vi "TRABAJO3.vi"() -> ()   [LabVIEW 2022 SP3]
panel:
  in  "Strings, Ciclos y Eventos":enum32{"EJERCICIO 1", "EJERCICIO 2"}(tab)
  out "SERIE FIBONACCI":string
  in  "LÍMITE SUPERIOR":dbl
  in  "?":bool
  out "ITERACIONES":dbl
  out "CONTADOR":dbl
  in  "?":bool
  in  "?":bool
  in  "?":bool
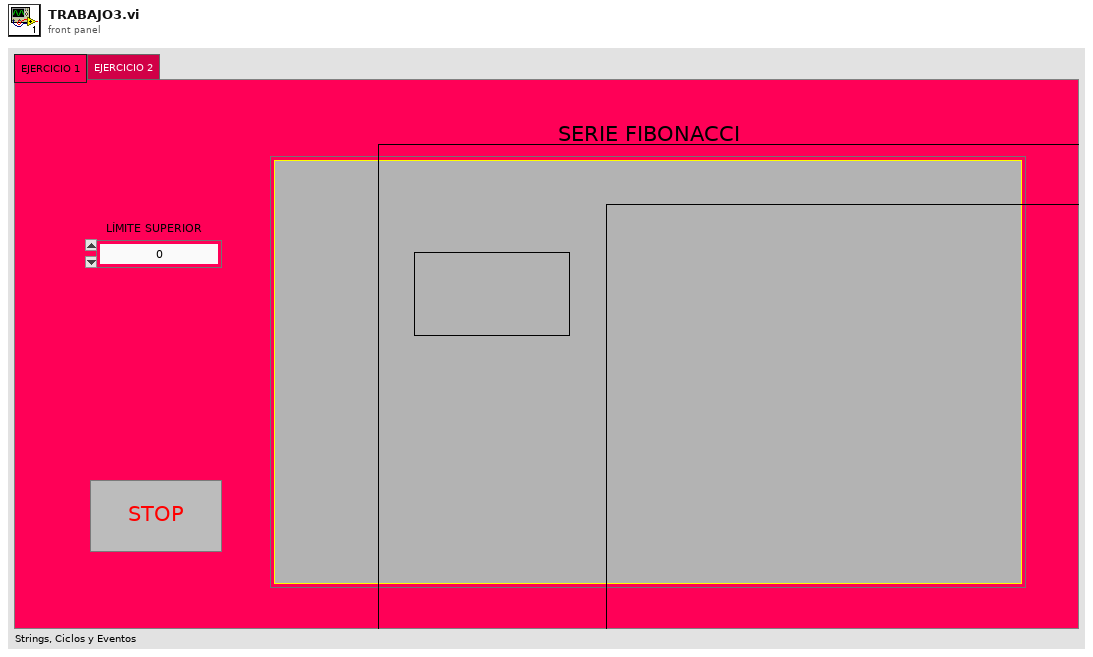
[diagram p1: front panel]
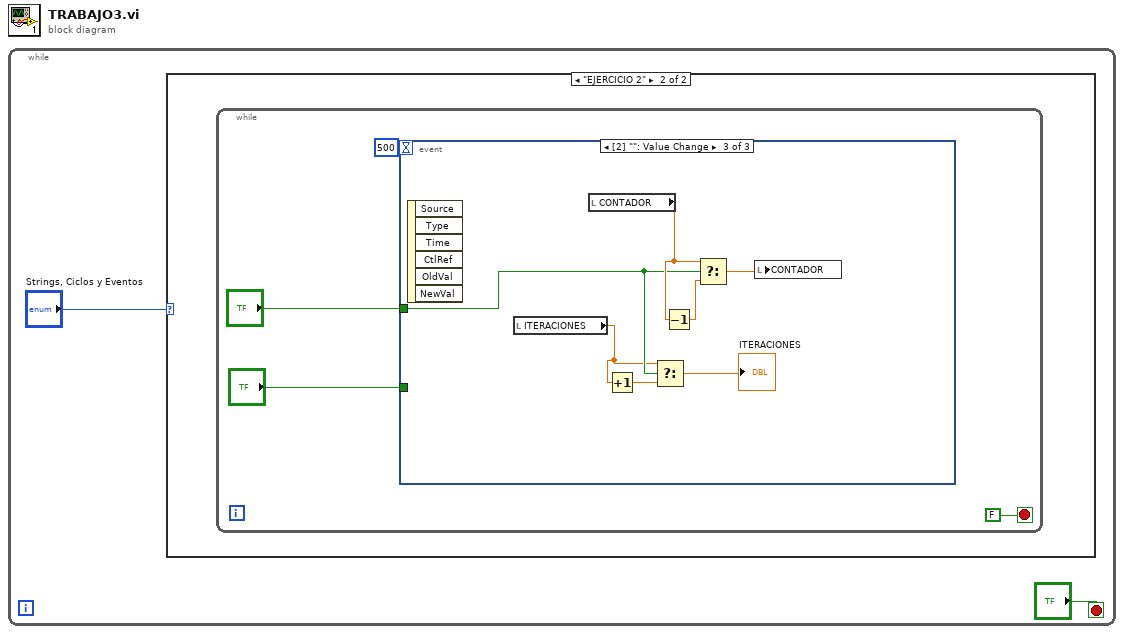
[diagram p0: block diagram]
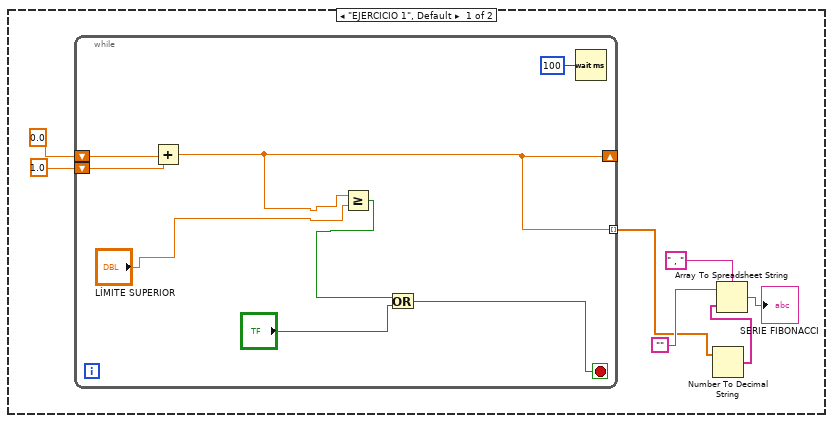
[diagram p2: hidden frame]
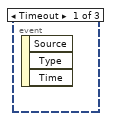
[diagram p3: hidden frame]
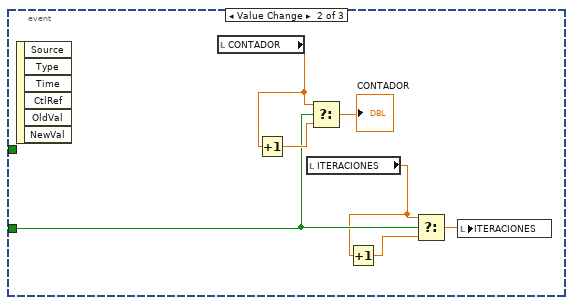
[diagram p4: hidden frame]
diagram:
  n1 = while {
    stop <- "?" stop-if-true
    n2 = case shown="\"EJERCICIO 2\"" "Strings, Ciclos y Eventos" {
      frame "EJERCICIO 1", Default {
        n3 = while {
          shift-right: [w12] -> _
          shift-left: 0.0 -> [w17]
          shift-left: 1.0 -> [w16]
          tunnel: [w12] -> w4 mode=indexing
          stop <- w14 stop-if-true
          n4 = Add(x=w17, y=w16) -> (x+y=w12:dbl)
          n5 = Greater Or Equal?(x=w12, y="LÍMITE SUPERIOR") -> (x >= y?=w10:bool)
          n6 = Or(x=w10, y="?") -> (x .or. y?=w14:bool)
          n7 = Wait (ms)(milliseconds to wait=u32 100) -> ()  [unwired: 1 out]
        }
        n8 = Number To Decimal String(number=w4) -> (decimal integer string=w3:string[])  [unwired: 1 in]
        n9 = Array To Spreadsheet String(delimiter (Tab)=" , ", array=w3, 3:"") -> (spreadsheet string=→"SERIE FIBONACCI":string)
      }
      frame "EJERCICIO 2" {
        n10 = while {
          stop <- FALSE stop-if-true
          n11 = event shown="[2] \"\": Value Change" {
            selector: _ -> [_ _ _]
            dyn-events: _ -> [_ _ _]
            timeout: 500 -> [_ _ _]
            tunnel: "?" -> [_ _ w31]
            tunnel: "?" -> [_ w24 _]
            event Timeout {
              n12 = event-data() -> ()  [unwired: 1 in, 3 out]
            }
            event Value Change {
              n13 = event-data() -> ()  [unwired: 1 in, 6 out]
              n14 = local read "CONTADOR"() -> (w26:dbl)
              n15 = Increment(x=w26) -> (x+1=w27:dbl)
              n16 = local read "ITERACIONES"() -> (w22:dbl)
              n17 = Select(t=w26, s=w24, f=w27) -> (s? t:f=→"CONTADOR":dbl)
              n18 = Increment(x=w22) -> (x+1=w23:dbl)
              n19 = Select(t=w22, s=w24, f=w23) -> (s? t:f=w25:dbl)
              n20 = local write "ITERACIONES"(w25) -> ()
            }
            event Value Change {
              n21 = event-data() -> ()  [unwired: 1 in, 6 out]
              n22 = local read "ITERACIONES"() -> (w29:dbl)
              n23 = local read "CONTADOR"() -> (w33:dbl)
              n24 = Increment(x=w29) -> (x+1=w30:dbl)
              n25 = Select(t=w29, s=w31, f=w30) -> (s? t:f=→"ITERACIONES":dbl)
              n26 = Decrement(x=w33) -> (x-1=w34:dbl)
              n27 = Select(t=w33, s=w31, f=w34) -> (s? t:f=w35:dbl)
              n28 = local write "CONTADOR"(w35) -> ()
            }
          }
        }
      }
    }
  }
